vi "Timeslot Arbiter.vi"(0 "write grant time (clocks)":u16=100, 5 "read grant time (clocks)":u16=100) -> (4 "write":bool, 6 "read":bool)   [LabVIEW 2012, in "FIFO.lvlib" / "niRFRIO Memory 1.0.0 FPGA.lvlib"]
uses:
  <userlib>/FPGA Library/Code Development/DRAM/RF-RIO/Memory/1.0.0/FPGA/niRFRIO Memory 1.0.0 FPGA.lvlib
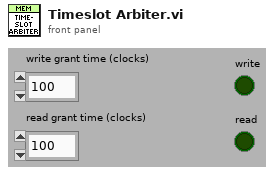
[diagram p1: front panel]
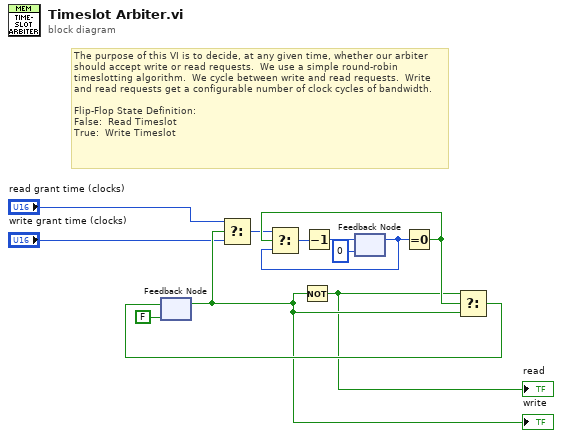
[diagram p0: block diagram]
diagram:
  # "The purpose of this VI is to decide, at any given time, whether our arbiter should accept write or read requests.  We use a simple round-robin timeslotting algorithm.  We cycle between write and read requests.  Write and read requests get a configurable number of clock cycles of bandwidth.\n\nFlip-Flop State Definition:\nFalse:  Read Timeslot\nTrue:  Write Timeslot"
  n1 = feedback #1 ("Cmd\nTimeslot")(FALSE ("read")) -> (w5:bool)
  "write" <- w5
  n2 = Select(t="read grant time (clocks)", s=w5, f="write grant time (clocks)") -> (s? t:f=w6:u16)
  n3 = Not(x=w5) -> (.not. x?=w3:bool)
  "read" <- w3
  n4 = feedback #2(u16 0) -> (w10:u16)
  n5 = Equal To 0?(x=w10) -> (x = 0?=w7:bool)
  n6 = Select(t=w6, s=w7, f=w10) -> (s? t:f=w9:u16)
  n7 = Decrement(x=w9) -> (x-1=w8:u16)
  n8 = feedback-in #2(w8) -> ()
  n9 = Select(t=w3, s=w7, f=w5) -> (s? t:f=w11:bool)
  n10 = feedback-in #1(w11) -> ()
